vi "set_image_params.vi"(8 "error in (no error)":errorcluster, 9 "iNbOfBuffer":u64, 10 "iImageHeight":u64, 11 "hCamera":u64) -> (0 "error out":errorcluster, 2 "hCamera":u64, 3 "function return":i32)   [LabVIEW 2013, in "Octoplus_LIDAR.lvlib"]
uses:
  <userlib>/Octoplus_LIDAR/Octoplus_LIDAR.lvlib
  <userlib>/Octoplus_LIDAR/CamCmosOctUsb3.dll
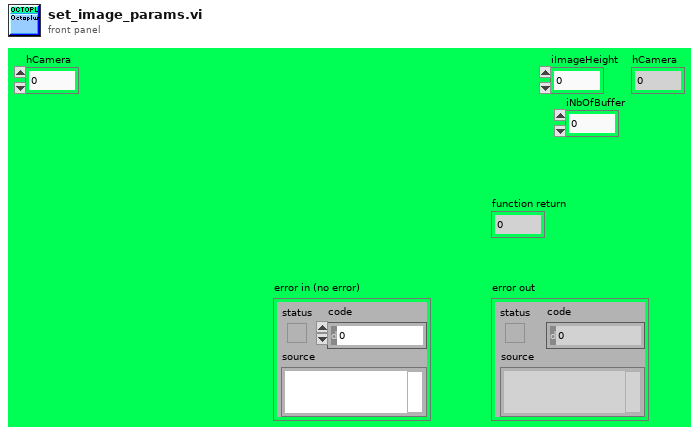
[diagram p1: front panel]
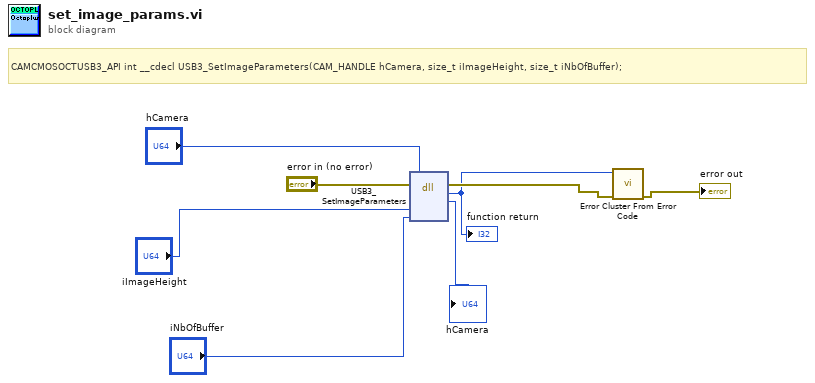
[diagram p0: block diagram]
diagram:
  # "CAMCMOSOCTUSB3_API int __cdecl USB3_SetImageParameters(CAM_HANDLE hCamera, size_t iImageHeight, size_t iNbOfBuffer);"
  n1 = dll-call lib="C:/Program Files/National Instruments/LabVIEW 2013/user.lib/Octoplus_LIDAR/CamCmosOctUsb3.dll" fn="USB3_SetImageParameters"(error in="error in (no error)", "hCamera"="hCamera", "iImageHeight"="iImageHeight", "iNbOfBuffer"="iNbOfBuffer") -> (error out=w3:errorcluster, "return type"=w1:i32, "hCamera"=→"hCamera":u64)  [unwired: 4 in, 1 out]
  "function return" <- w1
  n2 = call <vilib>:"Error Cluster From Error Code.vi"("error in (no error)"=w3, "error code (0)"=w1) -> ("error out"=→"error out":errorcluster)  [unwired: 7 in]
